vi "BuildSlideOGL.vi"(2 "Translation":cluster{"X":sgl, "Y":sgl, "Z":sgl}, 3 "Parameters":T1, 4 "slide":path, 5 "Stage In":refnum<vi>) -> (0 "Slide path":path, 1 "Stage out":refnum<vi>)   [LabVIEW 2010]
uses:
  ParamterCluster.ctl
  <vilib>/picture/3D Picture Control/NI_3D Picture Control.lvlib
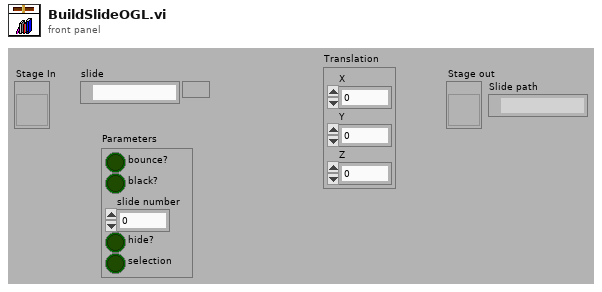
[diagram p1: front panel]
types:
  T1 = typedef "ParamterCluster.ctl" = cluster{"bounce?":bool, "black?":bool, "slide number":i32, "hide?":bool, "selection":bool}
  T2 = cluster{"X":sgl, "Y":sgl, "Z":sgl, "Color Box":u32, "Alpha":sgl}
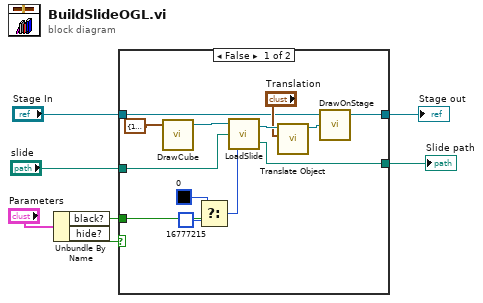
[diagram p0: block diagram]
diagram:
  n1 = Unbundle By Name("Parameters") -> ("black?"=w3:bool, "hide?"=w1:bool)
  n2 = case shown="False" w1 {
    tunnel: [w19 w21] -> w7
    tunnel: "slide" -> [w16 w21]
    tunnel: [w13 w22] -> w5
    tunnel: "Stage In" -> [w12 w22]
    tunnel: w3 -> [w11 _]
    frame False {
      n3 = call <userlib>:"DrawCube.vi"("Cube"=T2 {"X"=1.0, "Y"=1.0, "Z"=0.01, "Color Box"=16766250, "Alpha"=1.0}) -> ("object out"=w17:refnum<vi>)  [unwired: 5 in, 1 out]
      n4 = Select(t=u32 0 ("color(black)"), s=w11, f=u32 16777215 ("color(black)")) -> (s? t:f=w8:u32)
      n5 = call "LoadSlide.vi"("slide background"=w8, "Slide path"=w16, "object in"=w17) -> ("Slide path"=w19:path, "object out"=w18:refnum<vi>)
      n6 = call <vilib>:"Translate Object.vi"("Translation"="Translation", "Scene.Object In"=w18) -> ("Scene.Object Out"=w14:refnum<vi>)  [unwired: 8 in, 1 out]
      n7 = call <userlib>:"DrawOnStage.vi"("object in"=w14, "Stage in"=w12) -> ("Stage out"=w13:refnum<vi>)  [unwired: 1 in, 2 out]
    }
    frame True {
    }
  }
  "Slide path" <- w7
  "Stage out" <- w5
